vi "SW_Set_Cage_and_Recording_Settings.vi"(2 "error in (no error)":errorcluster) -> (0 "error out":errorcluster)   [LabVIEW 2018]
uses:
  Controls/CTL_Filter_selector.ctl
  Controls/CTL_Cage_diameter.ctl
  <vilib>/Utility/miscctls.llb/LVPointTypeDef.ctl
  <vilib>/Utility/sysdir.llb/System Directory Type.ctl
  SW_Globals_2.2+.vi
panel:
  in  "Default path":path
  out "Previous parameters":T3={"Data filtering"={"Filter type"=enum."Savitzky-Golay", "Length"=31, "Order"=3}, "Cage diameter, mm"=180, "Bridge V. offset"=0.0, "Bridge H. offset"=0.0, "Bridge swap"=FALSE, "Twisted neck"=FALSE, "Name prefix"="Track", "Stop at"=0.0, "\"Stop at\" enabled"=FALSE, "Default path"=path ""} {"Data filtering"."Order" min=3 max=11 step=2; "Data filtering"."Length" min=5 max=301 step=2; "Cage diameter, mm" items=["180 mm"=180, "240 mm"=240, "290 mm"=290, "325 mm"=325, "327 mm"=327, "333 mm"=333]}
  in  "Cage diameter, mm":T2=180 items=["180 mm"=180, "240 mm"=240, "290 mm"=290, "325 mm"=325, "327 mm"=327, "333 mm"=333]
  in  "Data filtering":T1={"Filter type"=enum."Savitzky-Golay", "Length"=31, "Order"=3} {"Order" min=3 max=11 step=2; "Length" min=5 max=301 step=2}
  in  "\"Stop at\" enabled":bool caption="Enable"
  in  "Bridge H. offset":sgl caption="Bridge hor. offset" min=-70 max=70 step=0.1 format="%#.1g"
  in  "Bridge swap":bool
  in  "Bridge V. offset":sgl caption="Bridge offset" min=-70 max=70 step=1 format="%#.0g"
  in  "Twisted neck":bool
  in  "Name Prefix":string="Track" caption="Savename prefix"
  in  "Stop record at":dbl caption="Stop at" min=0.0 max=43200.0 step=60.0 format="%<%H:%M:%S>t"
  in  "Reset to defaults":bool
  in  "Undo":bool
  in  "Save Config":bool
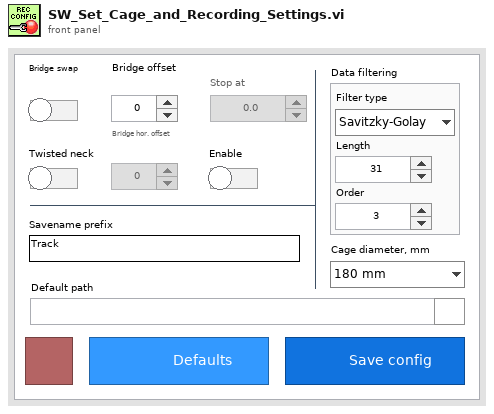
[diagram p1: front panel]
types:
  T1 = typedef "CTL_Filter_selector.ctl" = cluster{"Filter type":enum16{"None", "Savitzky-Golay"}, "Length":i32, "Order":i32}
  T2 = typedef "CTL_Cage_diameter.ctl" = u16
  T3 = cluster{"Data filtering":T1, "Cage diameter, mm":T2, "Bridge V. offset":sgl, "Bridge H. offset":sgl, "Bridge swap":bool, "Twisted neck":bool, "Name prefix":string, "Stop at":dbl, "\"Stop at\" enabled":bool, "Default path":path}
  T4 = typedef "LVPointTypeDef.ctl" = cluster{"Horizontal":i16, "Vertical":i16}
  T5 = typedef "CTL_Settings_cluster.ctl" = cluster{"Defaults":cluster{"Default User":dbl, "VISA Resource Name ":string}, "Recording and saving":cluster{"Researcher name":string, "Name prefix":string, "Data filtering":T1, "Stop at":dbl, "\"Stop at\" enabled":bool, "Default save folder path":path}, "Geometry":T6, "IO parameters":T7, "Stimulus presets array":T8[], "Settings loaded OK":bool}
  T6 = typedef "CTL_Segmented_plot_parameters.ctl" = cluster{"Cage diameter, mm":u16, "Starting angle MIDFIELD":i16, "Starting angle BORDER":i16, "Radius, mm CENTER":u16, "Radius, mm MIDFIELD":u16, "N segments MIDFIELD":u8, "N segments BORDER":u8, "R-gap, mm":sgl, "Bridge swap":bool, "Bridge H. offset":sgl, "Bridge V. offset":sgl, "Twisted neck":bool, "Alt. magn. orientation":bool}
  T7 = typedef "CTL_IO_params_cluster.ctl" = cluster{"IO general config.":u16, "IO 1 configuration":u16, "IO 2 configuration":u16, "IO 3 configuration":u16, "IO 4 configuration":u16, "Activate ext. RS-232":u16, "IO inversion config.":u16, "Sync capability":u8}
  T8 = typedef "CTL_Single_stimulus_setting.ctl" = cluster{"Event type":u16, "Dur., s":sgl, "Stim., s":sgl, "TTL out N":u16, "Set/Clear":bool, "Stim. has been set":bool}
  T9 = cluster{"Data filtering":T1, "Cage diameter, mm":u16, "Bridge V. offset":sgl, "Bridge H. offset":sgl, "Bridge swap":bool, "Twisted neck":bool, "Name prefix":string, "Stop at":dbl, "\"Stop at\" enabled":bool, "Default save folder path":path}
  T10 = enum8{"Enabled", "Disabled", "Disabled and Grayed Out"}
  T11 = typedef "System Directory Type.ctl" = i32
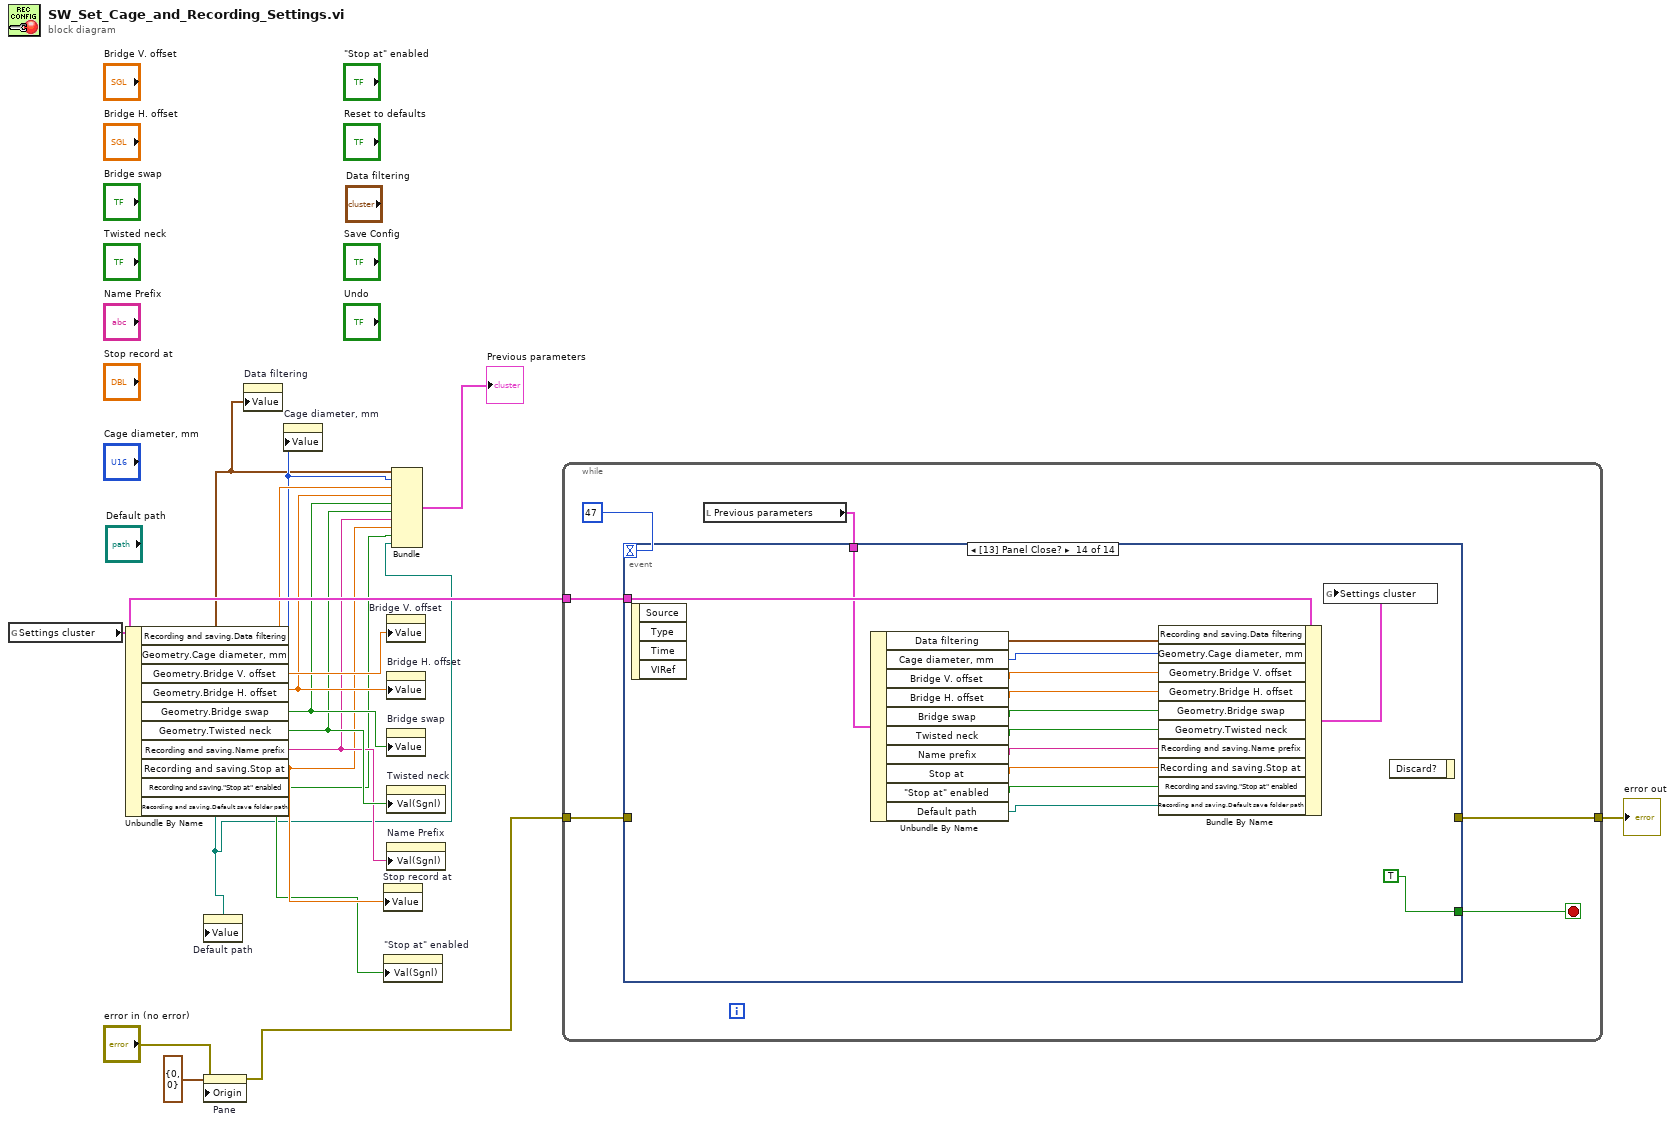
[diagram p0: block diagram]
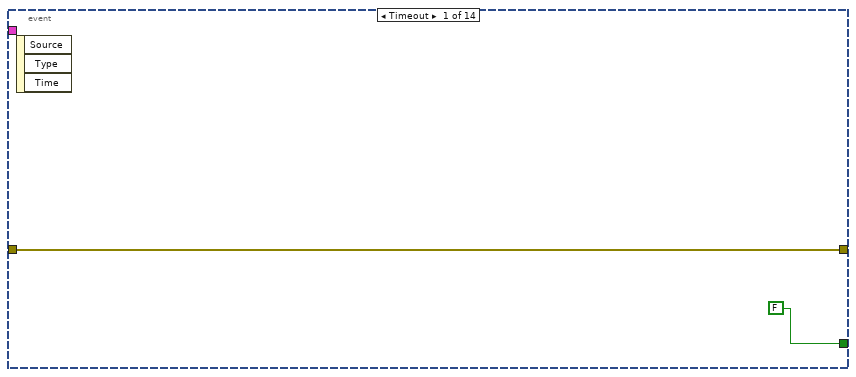
[diagram p2: hidden frame]
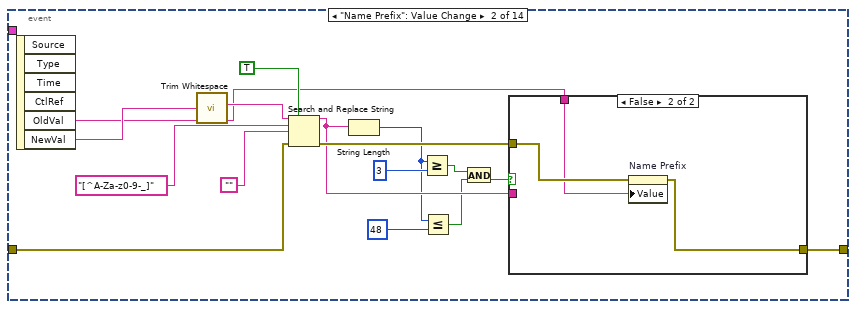
[diagram p3: hidden frame]
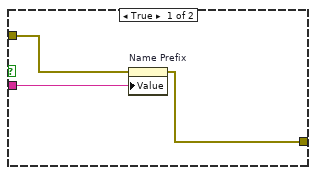
[diagram p4: hidden frame]
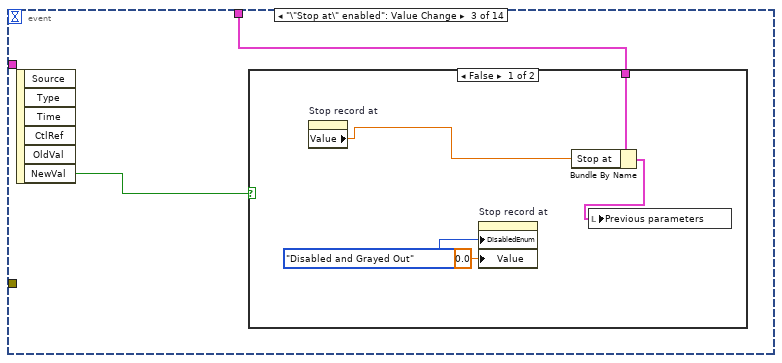
[diagram p5: hidden frame]
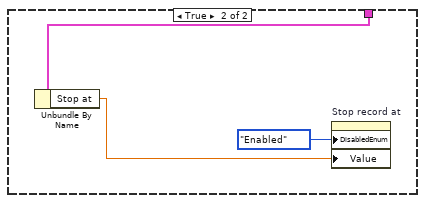
[diagram p6: hidden frame]
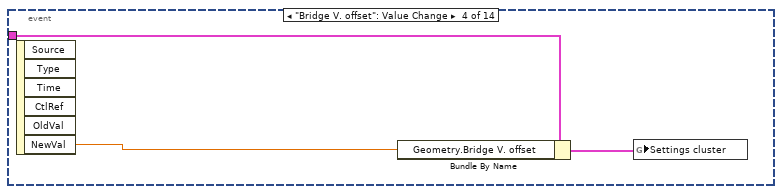
[diagram p7: hidden frame]
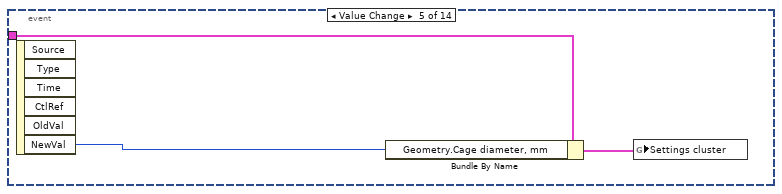
[diagram p8: hidden frame]
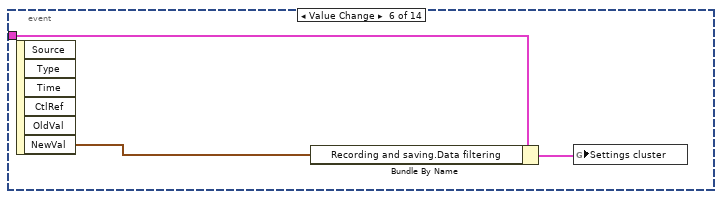
[diagram p9: hidden frame]
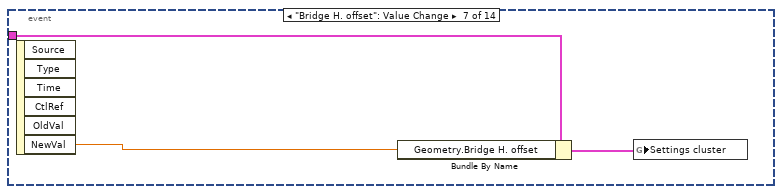
[diagram p10: hidden frame]
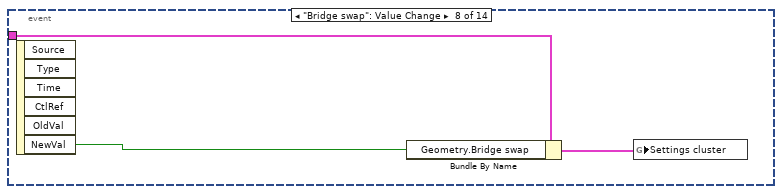
[diagram p11: hidden frame]
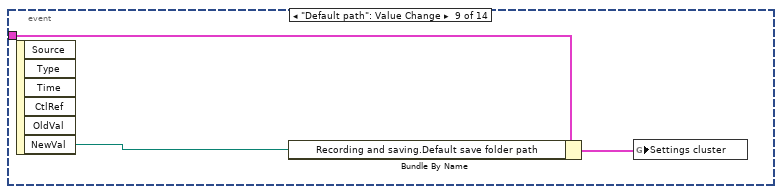
[diagram p12: hidden frame]
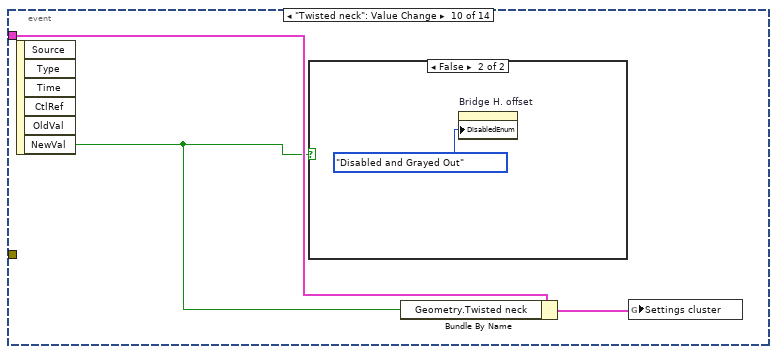
[diagram p13: hidden frame]
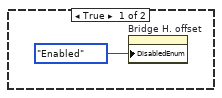
[diagram p14: hidden frame]
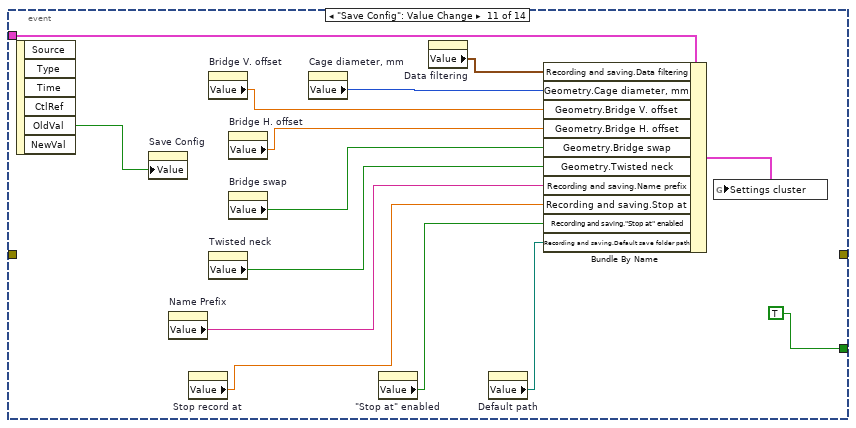
[diagram p15: hidden frame]
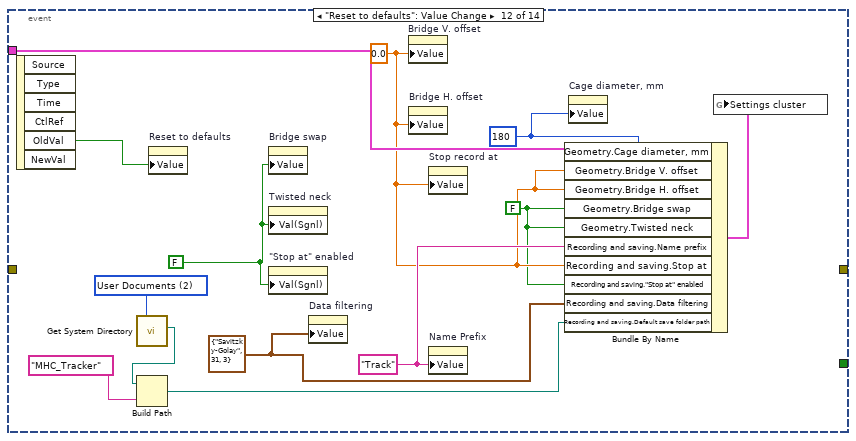
[diagram p16: hidden frame]
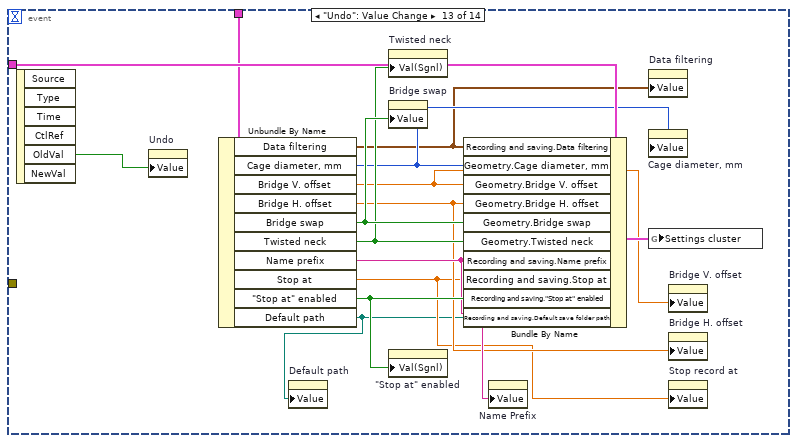
[diagram p17: hidden frame]
diagram:
  n1 = global read "SW_Globals_2.2+.vi" "Settings cluster"() -> (w15:T5)
  n2 = Unbundle By Name(w15) -> ("Recording and saving.Data filtering"=w2:T1, "Geometry.Cage diameter, mm"=w3:u16, "Geometry.Bridge V. offset"=w14:sgl, "Geometry.Bridge H. offset"=w13:sgl, "Geometry.Bridge swap"=w12:bool, "Geometry.Twisted neck"=w11:bool, "Recording and saving.Name prefix"=w10:string, "Recording and saving.Stop at"=w9:dbl, "Recording and saving.\"Stop at\" enabled"=w8:bool, "Recording and saving.Default save folder path"=w1:path)
  n3 = property on="Default path" class="Path"("Value"=w1) -> ()  [unwired: 2 in, 2 out]
  n4 = property on="Pane" class="Pane"(error in="error in (no error)", "Origin"=T4 {"Horizontal"=0, "Vertical"=0}) -> (error out=w5:errorcluster)  [unwired: 1 in, 1 out]
  n5 = property on="Data filtering" class="Clust (strict)"("Value"=w2) -> ()  [unwired: 2 in, 2 out]
  n6 = property on="Cage diameter, mm" class="Ring (strict)"("Value"=w3) -> ()  [unwired: 2 in, 2 out]
  n7 = property on="Stop record at" class="DigNum (strict)"("Value"=w9) -> ()  [unwired: 2 in, 2 out]
  n8 = property on="\"Stop at\" enabled" class="Bool (strict)"("Val(Sgnl)"=w8) -> ()  [unwired: 2 in, 2 out]
  n9 = property on="Bridge V. offset" class="DigNum (strict)"("Value"=w14) -> ()  [unwired: 2 in, 2 out]
  n10 = property on="Bridge H. offset" class="DigNum (strict)"("Value"=w13) -> ()  [unwired: 2 in, 2 out]
  n11 = property on="Bridge swap" class="Bool (strict)"("Value"=w12) -> ()  [unwired: 2 in, 2 out]
  n12 = property on="Twisted neck" class="Bool (strict)"("Val(Sgnl)"=w11) -> ()  [unwired: 2 in, 2 out]
  n13 = property on="Name Prefix" class="Str"("Val(Sgnl)"=w10) -> ()  [unwired: 2 in, 2 out]
  n14 = Bundle("Data filtering"=w2, "Cage diameter, mm"=w3, "Bridge V. offset"=w14, "Bridge H. offset"=w13, "Bridge swap"=w12, "Twisted neck"=w11, "Name prefix"=w10, "Stop at"=w9, "\"Stop at\" enabled"=w8, "Default save folder path"=w1) -> (→"Previous parameters":T9)  [unwired: 1 in]
  n15 = while {
    tunnel: w15 -> [w20]
    tunnel: w5 -> [w18]
    tunnel: [w19] -> w4
    stop <- w21 stop-if-true
    n16 = local read "Previous parameters"() -> (w17:T3)
    n17 = event shown="[13] Panel Close?" {
      selector: _ -> [_ _ _ _ _ _ _ _ _ _ _ _ _ _]
      dyn-events: _ -> [_ _ _ _ _ _ _ _ _ _ _ _ _ _]
      timeout: 47 -> [_ _ _ _ _ _ _ _ _ _ _ _ _ _]
      tunnel: [FALSE _ _ _ _ _ _ _ _ _ TRUE _ _ TRUE] -> w21
      tunnel: w20 -> [_ _ _ w59 w62 w64 w68 w71 w74 w76 w91 w104 w119 w133]
      tunnel: w17 -> [_ _ w47 _ _ _ _ _ _ _ _ _ w117 w131]
      tunnel: [w23 w25 _ _ _ _ _ _ _ _ _ _ _ _] -> w19
      tunnel: w18 -> [w23 w26 _ _ _ _ _ _ _ _ _ _ _ _]
      event Timeout {
        n18 = event-data() -> ()  [unwired: 1 in, 3 out]
      }
      event "Name Prefix": Value Change {
        n19 = event-data() -> ("OldVal"=w31:string, "NewVal"=w32:string)  [unwired: 1 in, 4 out]
        n20 = call <vilib>:"Trim Whitespace.vi"("string"=w32) -> ("trimmed string"=w38:string)  [unwired: 1 in]
        n21 = Search and Replace String(replace all?=TRUE ("replace all? (F)"), input string=w38, search string="[^A-Za-z0-9-_]" ("regular expression"), replace string="", error in=w26) -> (result string=w33:string, error out=w35:errorcluster)  [unwired: 3 in, 2 out]
        n22 = String Length(string=w33) -> (length=w30:i32)
        n23 = Greater Or Equal?(x=w30, y=3) -> (x >= y?=w34:bool)
        n24 = Less Or Equal?(x=w30, y=48) -> (x <= y?=w27:bool)
        n25 = And(x=w34, y=w27) -> (x .and. y?=w28:bool)
        n26 = case shown="False" w28 {
          tunnel: w35 -> [w43 w46]
          tunnel: w33 -> [w42 _]
          tunnel: w31 -> [_ w45]
          tunnel: [w41 w44] -> w25
          frame True {
            n27 = property on="Name Prefix" class="Str"(error in=w43, "Value"=w42) -> (error out=w41:errorcluster)  [unwired: 1 in, 1 out]
          }
          frame False {
            n28 = property on="Name Prefix" class="Str"(error in=w46, "Value"=w45) -> (error out=w44:errorcluster)  [unwired: 1 in, 1 out]
          }
        }
      }
      event "\"Stop at\" enabled": Value Change {
        n29 = event-data() -> ("NewVal"=w48:bool)  [unwired: 1 in, 5 out]
        n30 = case shown="False" w48 {
          tunnel: w47 -> [w51 w55]
          frame False {
            n31 = property on="Stop record at" class="DigNum (strict)"() -> ("Value"=w50:dbl)  [unwired: 2 in, 2 out]
            n32 = property on="Stop record at" class="DigNum (strict)"("DisabledEnum"=T10."Disabled and Grayed Out" ("Disabled"), "Value"=0.0 ("Stop record at")) -> ()  [unwired: 2 in, 2 out]
            n33 = Bundle By Name(cluster=w51, "Stop at"=w50) -> (w49:T3)
            n34 = local write "Previous parameters"(w49) -> ()
          }
          frame True {
            n35 = Unbundle By Name(w55) -> ("Stop at"=w54:dbl)
            n36 = property on="Stop record at" class="DigNum (strict)"("DisabledEnum"=T10."Enabled" ("Disabled"), "Value"=w54) -> ()  [unwired: 2 in, 2 out]
          }
        }
      }
      event "Bridge V. offset": Value Change {
        n37 = event-data() -> ("NewVal"=w58:sgl)  [unwired: 1 in, 5 out]
        n38 = Bundle By Name(cluster=w59, "Geometry.Bridge V. offset"=w58) -> (w57:T5)
        n39 = global write "SW_Globals_2.2+.vi" "Settings cluster"(w57) -> ()
      }
      event Value Change {
        n40 = event-data() -> ("NewVal"=w61:T2)  [unwired: 1 in, 5 out]
        n41 = Bundle By Name(cluster=w62, "Geometry.Cage diameter, mm"=w61) -> (w60:T5)
        n42 = global write "SW_Globals_2.2+.vi" "Settings cluster"(w60) -> ()
      }
      event Value Change {
        n43 = event-data() -> ("NewVal"=w63:T1)  [unwired: 1 in, 5 out]
        n44 = Bundle By Name(cluster=w64, "Recording and saving.Data filtering"=w63) -> (w65:T5)
        n45 = global write "SW_Globals_2.2+.vi" "Settings cluster"(w65) -> ()
      }
      event "Bridge H. offset": Value Change {
        n46 = event-data() -> ("NewVal"=w67:sgl)  [unwired: 1 in, 5 out]
        n47 = Bundle By Name(cluster=w68, "Geometry.Bridge H. offset"=w67) -> (w66:T5)
        n48 = global write "SW_Globals_2.2+.vi" "Settings cluster"(w66) -> ()
      }
      event "Bridge swap": Value Change {
        n49 = event-data() -> ("NewVal"=w70:bool)  [unwired: 1 in, 5 out]
        n50 = Bundle By Name(cluster=w71, "Geometry.Bridge swap"=w70) -> (w69:T5)
        n51 = global write "SW_Globals_2.2+.vi" "Settings cluster"(w69) -> ()
      }
      event "Default path": Value Change {
        n52 = event-data() -> ("NewVal"=w72:path)  [unwired: 1 in, 5 out]
        n53 = Bundle By Name(cluster=w74, "Recording and saving.Default save folder path"=w72) -> (w73:T5)
        n54 = global write "SW_Globals_2.2+.vi" "Settings cluster"(w73) -> ()
      }
      event "Twisted neck": Value Change {
        n55 = event-data() -> ("NewVal"=w75:bool)  [unwired: 1 in, 5 out]
        n56 = case shown="False" w75 {
          frame True {
            n57 = property on="Bridge H. offset" class="DigNum (strict)"("DisabledEnum"=T10."Enabled" ("Disabled")) -> ()  [unwired: 2 in, 2 out]
          }
          frame False {
            n58 = property on="Bridge H. offset" class="DigNum (strict)"("DisabledEnum"=T10."Disabled and Grayed Out" ("Disabled")) -> ()  [unwired: 2 in, 2 out]
          }
        }
        n59 = Bundle By Name(cluster=w76, "Geometry.Twisted neck"=w75) -> (w77:T5)
        n60 = global write "SW_Globals_2.2+.vi" "Settings cluster"(w77) -> ()
      }
      event "Save Config": Value Change {
        n61 = event-data() -> ("OldVal"=w92:bool)  [unwired: 1 in, 5 out]
        n62 = property on="Save Config" class="Bool (strict)"("Value"=w92) -> ()  [unwired: 2 in, 2 out]
        n63 = property on="Name Prefix" class="Str"() -> ("Value"=w86:string)  [unwired: 2 in, 2 out]
        n64 = property on="Stop record at" class="DigNum (strict)"() -> ("Value"=w85:dbl)  [unwired: 2 in, 2 out]
        n65 = property on="Bridge V. offset" class="DigNum (strict)"() -> ("Value"=w90:sgl)  [unwired: 2 in, 2 out]
        n66 = property on="Twisted neck" class="Bool (strict)"() -> ("Value"=w87:bool)  [unwired: 2 in, 2 out]
        n67 = property on="Bridge H. offset" class="DigNum (strict)"() -> ("Value"=w89:sgl)  [unwired: 2 in, 2 out]
        n68 = property on="Bridge swap" class="Bool (strict)"() -> ("Value"=w88:bool)  [unwired: 2 in, 2 out]
        n69 = property on="Cage diameter, mm" class="Ring (strict)"() -> ("Value"=w82:u16)  [unwired: 2 in, 2 out]
        n70 = property on="\"Stop at\" enabled" class="Bool (strict)"() -> ("Value"=w84:bool)  [unwired: 2 in, 2 out]
        n71 = property on="Data filtering" class="Clust (strict)"() -> ("Value"=w81:T1)  [unwired: 2 in, 2 out]
        n72 = property on="Default path" class="Path"() -> ("Value"=w80:path)  [unwired: 2 in, 2 out]
        n73 = Bundle By Name(cluster=w91, "Recording and saving.Data filtering"=w81, "Geometry.Cage diameter, mm"=w82, "Geometry.Bridge V. offset"=w90, "Geometry.Bridge H. offset"=w89, "Geometry.Bridge swap"=w88, "Geometry.Twisted neck"=w87, "Recording and saving.Name prefix"=w86, "Recording and saving.Stop at"=w85, "Recording and saving.\"Stop at\" enabled"=w84, "Recording and saving.Default save folder path"=w80) -> (w83:T5)
        n74 = global write "SW_Globals_2.2+.vi" "Settings cluster"(w83) -> ()
      }
      event "Reset to defaults": Value Change {
        w97 = T11 2 items=["User Home"=0, "User Desktop"=1, "User Documents"=2, "User Application Data"=3, "User Preferences"=4, "User Temporary"=5, "Public Documents"=6, "Public Application Data"=7, "Public Preferences"=8, "Public Cache"=13, "System Core Libraries"=9, "System Installed Libraries"=10, "Application Files"=11, "Boot Volume Root"=12] ("system directory type")
        w98 = T1 {"Filter type"=enum."Savitzky-Golay", "Length"=31, "Order"=3} ("Data filtering")
        w99 = u16 180 ("Geometry.Cage diameter, mm")
        w100 = FALSE ("Geometry.Bridge swap")
        w101 = sgl 0.0 ("Bridge offset")
        w102 = "Track" ("Value (Signaling)")
        w105 = FALSE
        n75 = event-data() -> ("OldVal"=w106:bool)  [unwired: 1 in, 5 out]
        n76 = call <vilib>:"Get System Directory.vi"("system directory type"=w97) -> ("system directory"=w96:path)  [unwired: 10 in]
        n77 = Build Path(base path=w96, name or relative path="MHC_Tracker") -> (appended path=w94:path)
        n78 = property on="Reset to defaults" class="Bool (strict)"("Value"=w106) -> ()  [unwired: 2 in, 2 out]
        n79 = property on="Bridge swap" class="Bool (strict)"("Value"=w105) -> ()  [unwired: 2 in, 2 out]
        n80 = property on="Twisted neck" class="Bool (strict)"("Val(Sgnl)"=w105) -> ()  [unwired: 2 in, 2 out]
        n81 = property on="\"Stop at\" enabled" class="Bool (strict)"("Val(Sgnl)"=w105) -> ()  [unwired: 2 in, 2 out]
        n82 = property on="Data filtering" class="Clust (strict)"("Value"=w98) -> ()  [unwired: 2 in, 2 out]
        n83 = property on="Bridge V. offset" class="DigNum (strict)"("Value"=w101) -> ()  [unwired: 2 in, 2 out]
        n84 = property on="Bridge H. offset" class="DigNum (strict)"("Value"=w101) -> ()  [unwired: 2 in, 2 out]
        n85 = property on="Stop record at" class="DigNum (strict)"("Value"=w101) -> ()  [unwired: 2 in, 2 out]
        n86 = property on="Name Prefix" class="Str"("Value"=w102) -> ()  [unwired: 2 in, 2 out]
        n87 = Bundle By Name(cluster=w104, "Geometry.Cage diameter, mm"=w99, "Geometry.Bridge V. offset"=w101, "Geometry.Bridge H. offset"=w101, "Geometry.Bridge swap"=w100, "Geometry.Twisted neck"=w100, "Recording and saving.Name prefix"=w102, "Recording and saving.Stop at"=w101, "Recording and saving.\"Stop at\" enabled"=w100, "Recording and saving.Data filtering"=w98, "Recording and saving.Default save folder path"=w94) -> (w103:T5)
        n88 = property on="Cage diameter, mm" class="Ring (strict)"("Value"=w99) -> ()  [unwired: 2 in, 2 out]
        n89 = global write "SW_Globals_2.2+.vi" "Settings cluster"(w103) -> ()
      }
      event "Undo": Value Change {
        n90 = event-data() -> ("OldVal"=w120:bool)  [unwired: 1 in, 5 out]
        n91 = property on="Undo" class="Bool (strict)"("Value"=w120) -> ()  [unwired: 2 in, 2 out]
        n92 = Unbundle By Name(w117) -> ("Data filtering"=w108:T1, "Cage diameter, mm"=w109:T2, "Bridge V. offset"=w112:sgl, "Bridge H. offset"=w111:sgl, "Bridge swap"=w116:bool, "Twisted neck"=w115:bool, "Name prefix"=w113:string, "Stop at"=w110:dbl, "\"Stop at\" enabled"=w114:bool, "Default path"=w107:path)
        n93 = property on="Default path" class="Path"("Value"=w107) -> ()  [unwired: 2 in, 2 out]
        n94 = property on="Twisted neck" class="Bool (strict)"("Val(Sgnl)"=w115) -> ()  [unwired: 2 in, 2 out]
        n95 = property on="Bridge swap" class="Bool (strict)"("Value"=w116) -> ()  [unwired: 2 in, 2 out]
        n96 = property on="\"Stop at\" enabled" class="Bool (strict)"("Val(Sgnl)"=w114) -> ()  [unwired: 2 in, 2 out]
        n97 = Bundle By Name(cluster=w119, "Recording and saving.Data filtering"=w108, "Geometry.Cage diameter, mm"=w109, "Geometry.Bridge V. offset"=w112, "Geometry.Bridge H. offset"=w111, "Geometry.Bridge swap"=w116, "Geometry.Twisted neck"=w115, "Recording and saving.Name prefix"=w113, "Recording and saving.Stop at"=w110, "Recording and saving.\"Stop at\" enabled"=w114, "Recording and saving.Default save folder path"=w107) -> (w118:T5)
        n98 = property on="Name Prefix" class="Str"("Value"=w113) -> ()  [unwired: 2 in, 2 out]
        n99 = property on="Data filtering" class="Clust (strict)"("Value"=w108) -> ()  [unwired: 2 in, 2 out]
        n100 = property on="Cage diameter, mm" class="Ring (strict)"("Value"=w109) -> ()  [unwired: 2 in, 2 out]
        n101 = global write "SW_Globals_2.2+.vi" "Settings cluster"(w118) -> ()
        n102 = property on="Bridge V. offset" class="DigNum (strict)"("Value"=w112) -> ()  [unwired: 2 in, 2 out]
        n103 = property on="Bridge H. offset" class="DigNum (strict)"("Value"=w111) -> ()  [unwired: 2 in, 2 out]
        n104 = property on="Stop record at" class="DigNum (strict)"("Value"=w110) -> ()  [unwired: 2 in, 2 out]
      }
      event Panel Close? {
        n105 = event-data() -> ()  [unwired: 1 in, 4 out]
        n106 = Unbundle By Name(w131) -> ("Data filtering"=w122:T1, "Cage diameter, mm"=w123:T2, "Bridge V. offset"=w130:sgl, "Bridge H. offset"=w129:sgl, "Bridge swap"=w128:bool, "Twisted neck"=w127:bool, "Name prefix"=w126:string, "Stop at"=w125:dbl, "\"Stop at\" enabled"=w124:bool, "Default path"=w121:path)
        n107 = Bundle By Name(cluster=w133, "Recording and saving.Data filtering"=w122, "Geometry.Cage diameter, mm"=w123, "Geometry.Bridge V. offset"=w130, "Geometry.Bridge H. offset"=w129, "Geometry.Bridge swap"=w128, "Geometry.Twisted neck"=w127, "Recording and saving.Name prefix"=w126, "Recording and saving.Stop at"=w125, "Recording and saving.\"Stop at\" enabled"=w124, "Recording and saving.Default save folder path"=w121) -> (w132:T5)
        n108 = global write "SW_Globals_2.2+.vi" "Settings cluster"(w132) -> ()
        n109 = event-data() -> ()  [unwired: 2 in, 1 out]
      }
    }
  }
  "error out" <- w4
